vi "servo_orig.vi"() -> ()   [LabVIEW 2014]
uses:
  <vilib>/myRIO/Instrument Drivers/Onboard IO/PWM/typedefs/PWM Reference.ctl
  <vilib>/myRIO/Common/Instrument Driver Framework/Utilities/typedefs/myRIO Generic Hardware Reference.ctl
  <vilib>/myRIO/Common/Instrument Driver Framework/Utilities/typedefs/Hardware Version Enum.ctl
  <vilib>/myRIO/Common/Instrument Driver Framework/Utilities/typedefs/myRIO v1.0 Reference.ctl
  <vilib>/myRIO/Common/Instrument Driver Framework/Utilities/typedefs/Generic FPGA Reference.ctl
  <vilib>/myRIO/Common/Instrument Driver Framework/myRIO v1.0/PWM/typedefs/PWM Channels Enum.ctl
  <vilib>/myRIO/Instrument Drivers/Onboard IO/PWM/typedefs/PWM Configuration.ctl
  <vilib>/userdefined/High Color/nirio_resource_hc.ctl
  <vilib>/myRIO/Common/Instrument Driver Framework/myRIO v1.0/PWM/vis/myRIO v1.1 Open PWM.vi
  <vilib>/myRIO/Common/Instrument Driver Framework/Utilities/vis/Validate Channels.vi
  <vilib>/myRIO/Common/Instrument Driver Framework/myRIO v1.0/PWM/vis/myRIO v1.0 Reserve PWM.vi
  <vilib>/myRIO/Instrument Drivers/Onboard IO/PWM/vis/Set Duty Cycle and Frequency.vi
  <vilib>/myRIO/Common/Instrument Driver Framework/myRIO v1.0/DIO/vis/myRIO v1.1 Open DIO.vi
  <vilib>/myRIO/Common/Instrument Driver Framework/myRIO v1.0/PWM/vis/myRIO v1.0 Close PWM.vi
  <vilib>/myRIO/Common/Instrument Driver Framework/myRIO v1.0/DIO/vis/myRIO v1.0 Close DIO.vi
  <vilib>/myRIO/Common/Instrument Driver Framework/myRIO v1.0/PWM/vis/myRIO v1.0 Build MUX Configuration PWM.vi
  <vilib>/myRIO/Common/Instrument Driver Framework/myRIO v1.0/Resource Manager/vis/myRIO v1.0 Reserve Channel List.vi
  <vilib>/myRIO/Common/Instrument Driver Framework/myRIO v1.0/DIO/vis/myRIO v1.0 Reserve DIO.vi
  <vilib>/myRIO/Common/Instrument Driver Framework/myRIO v1.0/PWM/vis/myRIO v1.0 Unreserve PWM.vi
  <vilib>/myRIO/Common/Instrument Driver Framework/myRIO v1.0/DIO/vis/myRIO v1.0 Unreserve DIO.vi
  <vilib>/myRIO/Common/Instrument Driver Framework/myRIO v1.0/Resource Manager/vis/myRIO v1.0 Create Configuration List.vi
  <vilib>/myRIO/Common/Instrument Driver Framework/myRIO v1.0/Resource Manager/vis/myRIO v1.0 Reserve Channel.vi
  <vilib>/myRIO/Common/Instrument Driver Framework/myRIO v1.0/Resource Manager/vis/myRIO v1.0 Unreserve Channel.vi
  <vilib>/myRIO/Common/Instrument Driver Framework/myRIO v1.0/DIO/vis/myRIO v1.0 Build MUX Configuration DIO.vi
  <vilib>/myRIO/Common/Instrument Driver Framework/myRIO v1.0/Resource Manager/vis/myRIO v1.0 Unreserve Channel List.vi
  <vilib>/myRIO/Common/Instrument Driver Framework/myRIO v1.0/Resource Manager/vis/myRIO v1.0 Build Mutex Name.vi
  <vilib>/Utility/VariantDataType/GetNumericInfo.vi
  <vilib>/Utility/error.llb/Error Cluster From Error Code.vi
  <vilib>/myRIO/Common/Instrument Driver Framework/myRIO v1.0/myRIO v1.1 Open.vi
  <vilib>/myRIO/Common/Instrument Driver Framework/Utilities/vis/IO Manager.vi
  <vilib>/myRIO/Common/Instrument Driver Framework/Utilities/vis/Configuration Manager.vi
  <vilib>/myRIO/Common/Instrument Driver Framework/myRIO v1.0/Resource Manager/vis/myRIO v1.0 Configure IO.vi
  <vilib>/myRIO/Common/Instrument Driver Framework/myRIO v1.0/myRIO v1.0 Close.vi
  <vilib>/myRIO/Common/Instrument Driver Framework/myRIO v1.0/PWM/vis/myRIO v1.0 Write PWM.vi
  <vilib>/myRIO/Common/Instrument Driver Framework/myRIO v1.0/PWM/vis/myRIO v1.0 Shutdown PWM.vi
  <vilib>/myRIO/Common/Instrument Driver Framework/myRIO v1.0/DIO/vis/myRIO v1.0 Write DIO.vi
  <vilib>/myRIO/Common/Instrument Driver Framework/myRIO v1.0/DIO/vis/myRIO v1.0 Shutdown DIO.vi
  <vilib>/myRIO/Instrument Drivers/Onboard IO/PWM/vis/myRIO PWM Open.xnode
  <vilib>/myRIO/Instrument Drivers/Onboard IO/DIO/DIO.lvlib
  <vilib>/myRIO/Instrument Drivers/Onboard IO/PWM/PWM.lvlib
panel:
  in  "Channel Name":tag="C/PWM0"
  in  "Servo Position":dbl(slide)=1500.0 scale=500.0..2500.0
  out "error out":errorcluster
  out "Active":bool
  in  "Stop":bool
  # "This VI reads the voltage value of a potentiometer"
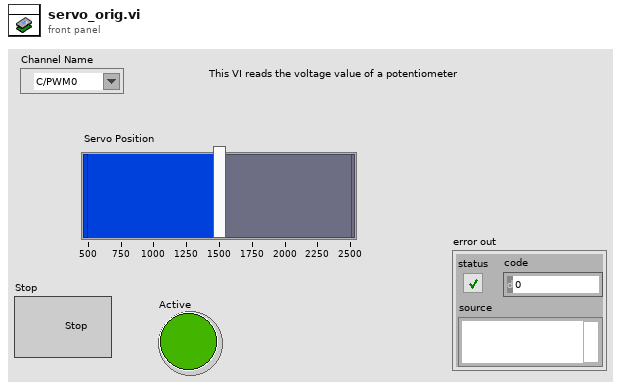
[diagram p1: front panel]
types:
  T1 = typedef "nirio_resource_hc.ctl" = tag
  T2 = typedef "Hardware Version Enum.ctl" = enum16{"Unknown", "myRIO-1900", "myRIO-1950"}
  T3 = typedef "PWM.lvlib/PWM Reference.ctl" = cluster{"myRIO Reference":T4, "PWM Channels Enum":T7, "PWM Configuration":T8}
  T4 = typedef "myRIO Generic Hardware Reference.ctl" = cluster{"myRIO Model":T2, "myRIO Hardware Reference":T5}
  T5 = typedef "myRIO v1.0 Reference.ctl" = cluster{"Generic FPGA Reference":T6, "Allow multiple opens":bool}
  T6 = typedef "Generic FPGA Reference.ctl" = refnum<k20>
  T7 = typedef "PWM Channels Enum.ctl" = enum16{"Not Connected", "C/PWM0", "C/PWM1", "A/PWM0", "A/PWM1", "A/PWM2", "B/PWM0", "B/PWM1", "B/PWM2"}
  T8 = typedef "PWM.lvlib/PWM Configuration.ctl" = cluster{"Frequency":dbl, "Duty Cycle":dbl}
  T9 = typedef "DIO.lvlib/DIO Reference.ctl" = cluster{"myRIO Reference":T4, "DIO Channels List":T10}
  T10 = typedef "DIO Channels List.ctl" = T11[]
  T11 = typedef "DIO Channels Enum.ctl" = enum16{"Not Connected", "C/DIO0", "C/DIO1", "C/DIO2", "C/DIO3", "C/DIO4", "C/DIO5", "C/DIO6", "C/DIO7", "A/DIO0", "A/DIO1", "A/DIO2", "A/DIO3", "A/DIO4", "A/DIO5", "A/DIO6", "A/DIO7", "A/DIO8", "A/DIO9", "A/DIO10", "A/DIO11", "A/DIO12", "A/DIO13", "A/DIO14", "A/DIO15", "B/DIO0", "B/DIO1", "B/DIO2", "B/DIO3", "B/DIO4", "B/DIO5", "B/DIO6", "B/DIO7", "B/DIO8", "B/DIO9", "B/DIO10", "B/DIO11", "B/DIO12", "B/DIO13", "B/DIO14", "B/DIO15", "LED0", "LED1", "LED2", "LED3", "Button0"}
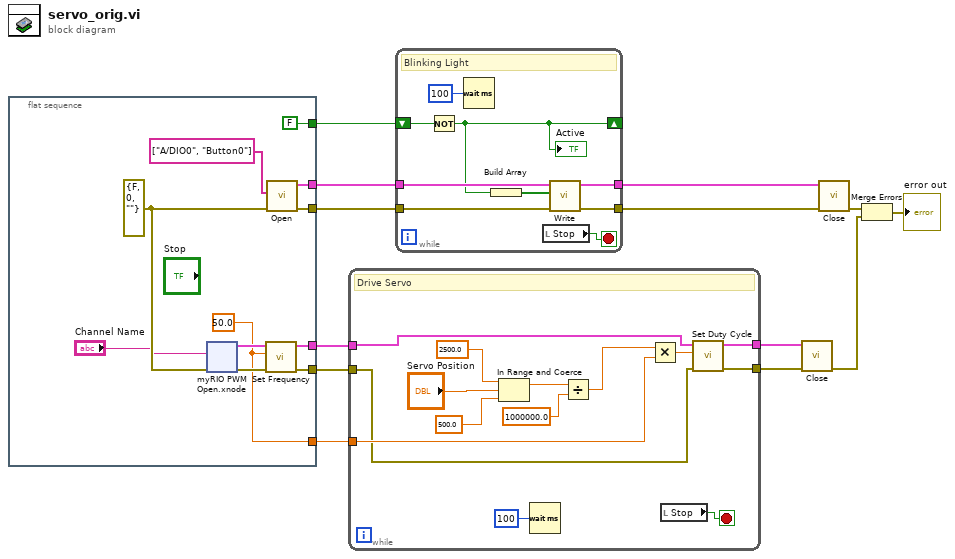
[diagram p0: block diagram]
diagram:
  n1 = flat-sequence {
    tunnel: [w23] -> w12
    tunnel: [w22] -> w11
    tunnel: [FALSE] -> w13
    tunnel: [w16] -> w9
    tunnel: [w17] -> w10
    tunnel: [w15] -> w4
    frame #0 {
      w15 = 50.0 ("Frequency [Hz]")
      w18 = errorcluster {"status"=FALSE, "code"=0, "source"=""} ("error out")
      n2 = xnode "myRIO PWM Open.xnode"("error in (no error)"=w18, "Channel Name"="Channel Name") -> ("error out"=w20:errorcluster, "PWM Ref Out"=w19:T3)  [unwired: 1 in]
      n3 = call <vilib>:"Set Frequency.vi"("error in (no error)"=w20, "Frequency [Hz]"=w15, "PWM Ref In"=w19) -> ("error out"=w16:errorcluster, "PWM Ref Out"=w17:T3)  [unwired: 6 in]
      n4 = call <vilib>:"Open.vi"("error in (no error)"=w18, "Channel Names"=tag[] ["A/DIO0", "Button0"]) -> ("error out"=w22:errorcluster, "DIO Ref Out"=w23:T9)  [unwired: 8 in]
    }
  }
  n5 = while {
    tunnel: w10 -> [w45]
    tunnel: w9 -> [w42]
    tunnel: w4 -> [w47]
    tunnel: [w44] -> w1
    tunnel: [w43] -> w2
    stop <- w54 stop-if-true
    # "Drive Servo"
    n6 = In Range and Coerce(upper limit=2500.0, x="Servo Position", lower limit=500.0) -> (coerced(x)=w50:dbl)  [unwired: 1 out]
    n7 = Wait (ms)(milliseconds to wait=u32 100) -> ()  [unwired: 1 out]
    n8 = Divide(x=w50, y=1000000.0) -> (x/y=w48:dbl)
    n9 = Multiply(x=w48, y=w47) -> (x*y=w46:dbl)
    n10 = local read "Stop"() -> (w54:bool)
    n11 = call <vilib>:"Set Duty Cycle.vi"("error in (no error)"=w42, "Duty Cycle"=w46, "PWM Ref In"=w45) -> ("error out"=w43:errorcluster, "PWM Ref Out"=w44:T3)  [unwired: 6 in]
  }
  n12 = while {
    shift-right: [w55] -> _
    shift-left: w13 -> [w61]
    tunnel: w12 -> [w59]
    tunnel: w11 -> [w58]
    tunnel: [w57] -> w7
    tunnel: [w56] -> w8
    stop <- w62 stop-if-true
    # "Blinking Light"
    n13 = Not(x=w61) -> (.not. x?=w55:bool)
    "Active" <- w55
    n14 = Wait (ms)(milliseconds to wait=u32 100) -> ()  [unwired: 1 out]
    n15 = Build Array(w55) -> (w60:bool[])
    n16 = local read "Stop"() -> (w62:bool)
    n17 = call <vilib>:"Write.vi"("error in (no error)"=w58, "Values"=w60, "DIO Ref In"=w59) -> ("error out"=w57:errorcluster, "DIO Ref Out"=w56:T9)  [unwired: 6 in]
  }
  n18 = call <vilib>:"Close.vi"("error in (no error)"=w2, "PWM Ref In"=w1) -> ("error out"=w3:errorcluster)  [unwired: 9 in]
  n19 = call <vilib>:"Close.vi"("error in (no error)"=w7, "DIO Ref In"=w8) -> ("error out"=w6:errorcluster)  [unwired: 9 in]
  n20 = Merge Errors(w6, w3) -> (→"error out":errorcluster)
